vi "LEBITplc.ParseDBArray.vi"(1 "DBArray":string[][](array[string])) -> (9 "PLC?":bool[](array[boolean]), 10 "nickname":string[](array[string]), 11 "SetValue":dbl[][](array[numeric]), 12 "monValuePLC":string[](array[string]), 13 "MonValueServiceID":i32[](array[numeric]), 14 "setValuePLC":string[](array[string]), 15 "BaseNames":string[](array[string]), 16 "MonitorDependent":string[](array[string]), 17 "Special":string[](array[string]), 18 "setValuePLCServiceID":i32[](array[numeric]), 19 "SetValueServiceID":i32[](array[numeric]))   [LabVIEW 2014, in "LEBITplc.lvlib"]
uses:
  LEBITplc.lvlib
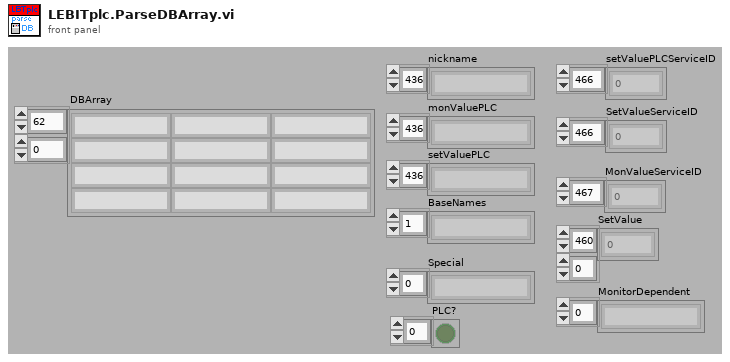
[diagram p1: front panel]
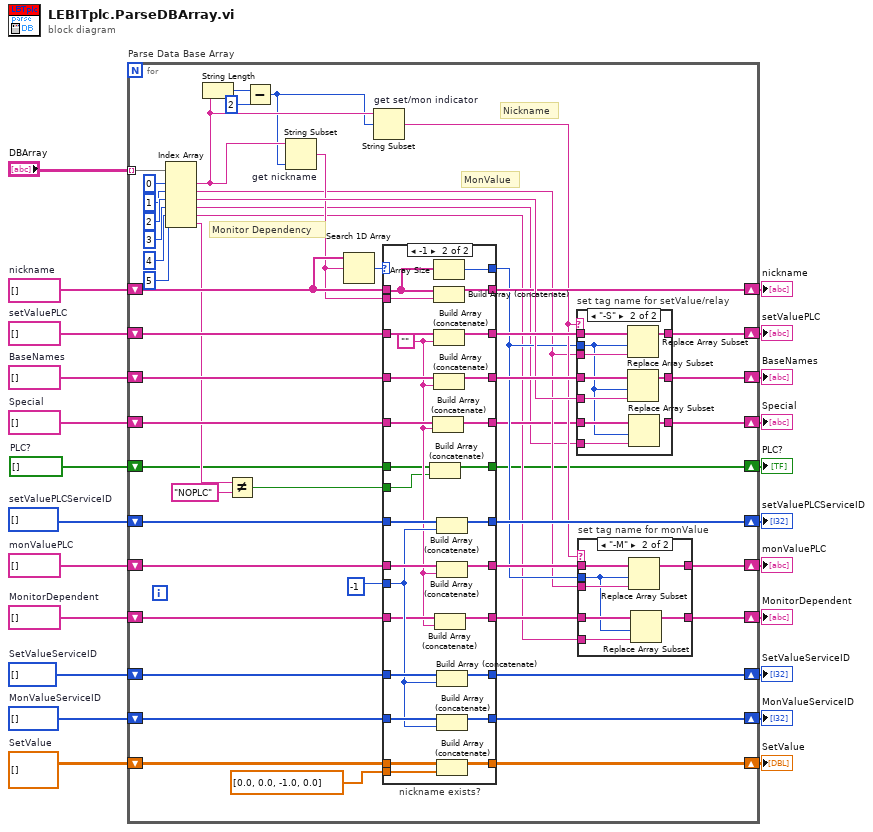
[diagram p0: block diagram]
diagram:
  w2 = bool[] []  # PLC?
  w4 = string[] []  # Special
  w6 = string[] []  # MonitorDependent
  w8 = dbl[][] []  # SetValue
  w18 = i32[] []  # MonValueServiceID
  w19 = i32[] []  # SetValueServiceID
  w20 = string[] []  # monValuePLC
  w17 = i32[] []  # setValuePLCServiceID
  w21 = string[] []  # BaseNames
  w22 = string[] []  # setValuePLC
  w23 = string[] []  # nickname
  n1 = for "Parse Data Base Array" {
    tunnel: "DBArray" -> [w74] mode=indexing
    shift-right: [w57] -> w16
    shift-left: w23 -> [w67]
    shift-right: [w56] -> w15
    shift-left: w22 -> [w66]
    shift-right: [w55] -> w14
    shift-left: w21 -> [w65]
    shift-right: [w53] -> w13
    shift-left: w17 -> [w54]
    shift-right: [w51] -> w12
    shift-left: w20 -> [w64]
    shift-right: [w50] -> w11
    shift-left: w19 -> [w63]
    shift-right: [w49] -> w10
    shift-left: w18 -> [w62]
    shift-right: [w46] -> w7
    shift-left: w8 -> [w47]
    shift-right: [w39] -> w5
    shift-left: w6 -> [w41]
    shift-right: [w33] -> w3
    shift-left: w4 -> [w35]
    shift-right: [w24] -> w1
    shift-left: w2 -> [w25]
    # "MonValue"
    # "Nickname"
    # "Monitor Dependency"
    n2 = Index Array(array=w74, index #1=0 ("index"), index #2=1 ("index"), index #3=2 ("index"), index #4=3 ("index"), index #5=4 ("index"), index #6=5 ("index")) -> (element #1=w70:string, element #2=w42:string, element #3=w58:string, element #4=w30:string, element #5=w31:string, element #6=w28:string)
    n3 = String Length(string=w70) -> (length=w72:i32)
    n4 = Not Equal?(x=w28, y="NOPLC") -> (x != y?=w26:bool)
    n5 = Subtract(x=w72, y=2) -> (x-y=w69:i32)
    n6 = String Subset "get nickname"(string=w70, length (rest)=w69) -> (substring=w44:string)  [unwired: 1 in]
    n7 = Search 1D Array(1D array=w67, element=w44) -> (index of element=w68:i32)  [unwired: 1 in]
    n8 = String Subset "get set/mon indicator"(string=w70, offset (0)=w69) -> (substring=w48:string)  [unwired: 1 in]
    n9 = case "nickname exists?" shown="-1" w68 {
      selector: w68 -> [w88 _]
      tunnel: w67 -> [w95 w110]
      tunnel: w44 -> [_ w123]
      tunnel: [w95 w122] -> w57
      tunnel: w66 -> [w94 w121]
      tunnel: w65 -> [w93 w120]
      tunnel: w54 -> [w92 w119]
      tunnel: w64 -> [w91 w118]
      tunnel: w63 -> [w90 w117]
      tunnel: w62 -> [w89 w116]
      tunnel: [w94 w115] -> w60
      tunnel: [w93 w114] -> w59
      tunnel: [w92 w111] -> w53
      tunnel: [w91 w112] -> w52
      tunnel: [w90 w113] -> w50
      tunnel: [w89 w107] -> w49
      tunnel: -1 -> [_ w104]
      tunnel: [w88 w109] -> w43
      tunnel: w47 -> [w87 w108]
      tunnel: dbl[] [0.0, 0.0, -1.0, 0.0] -> [_ w106]
      tunnel: [w87 w105] -> w46
      tunnel: w41 -> [w86 w103]
      tunnel: [w86 w102] -> w40
      tunnel: w35 -> [w85 w101]
      tunnel: [w85 w99] -> w34
      tunnel: w26 -> [_ w98]
      tunnel: w25 -> [w84 w97]
      tunnel: [w84 w96] -> w24
      frame 0, Default {
      }
      frame -1 {
        w100 = ""
        n10 = Build Array (concatenate)(w97, w98) -> (w96:bool[])
        n11 = Build Array (concatenate)(w101, w100) -> (w99:string[])
        n12 = Array Size(array=w110) -> (size(s)=w109:i32)
        n13 = Build Array (concatenate)(w110, w123) -> (w122:string[])
        n14 = Build Array (concatenate)(w121, w100) -> (w115:string[])
        n15 = Build Array (concatenate)(w120, w100) -> (w114:string[])
        n16 = Build Array (concatenate)(w103, w100) -> (w102:string[])
        n17 = Build Array (concatenate)(w119, w104) -> (w111:i32[])
        n18 = Build Array (concatenate)(w118, w100) -> (w112:string[])
        n19 = Build Array (concatenate)(w117, w104) -> (w113:i32[])
        n20 = Build Array (concatenate)(w116, w104) -> (w107:i32[])
        n21 = Build Array (concatenate)(w108, w106) -> (w105:dbl[][])
      }
    }
    n22 = case "set tag name for setValue/relay" shown="\"-S\"" w48 {
      tunnel: w60 -> [w126 w136]
      tunnel: w43 -> [_ w127]
      tunnel: w42 -> [_ w135]
      tunnel: w59 -> [w125 w132]
      tunnel: w58 -> [_ w131]
      tunnel: [w126 w134] -> w56
      tunnel: [w125 w133] -> w55
      tunnel: w34 -> [w124 w130]
      tunnel: [w124 w129] -> w33
      tunnel: w30 -> [_ w128]
      frame Default {
      }
      frame "-S" {
        n23 = Replace Array Subset(array=w136, new element=w135, index=w127) -> (w134:string[])
        n24 = Replace Array Subset(array=w132, new element=w131, index=w127) -> (w133:string[])
        n25 = Replace Array Subset(array=w130, new element=w128, index=w127) -> (w129:string[])
      }
    }
    n26 = case "set tag name for monValue" shown="\"-M\"" w48 {
      tunnel: w52 -> [w76 w83]
      tunnel: w43 -> [_ w78]
      tunnel: w42 -> [_ w82]
      tunnel: [w76 w81] -> w51
      tunnel: w40 -> [w75 w80]
      tunnel: [w75 w79] -> w39
      tunnel: w31 -> [_ w77]
      frame Default {
      }
      frame "-M" {
        n27 = Replace Array Subset(array=w83, new element=w82, index=w78) -> (w81:string[])
        n28 = Replace Array Subset(array=w80, new element=w77, index=w78) -> (w79:string[])
      }
    }
  }
  "nickname" <- w16
  "setValuePLC" <- w15
  "BaseNames" <- w14
  "setValuePLCServiceID" <- w13
  "monValuePLC" <- w12
  "SetValueServiceID" <- w11
  "MonValueServiceID" <- w10
  "SetValue" <- w7
  "MonitorDependent" <- w5
  "Special" <- w3
  "PLC?" <- w1
